vi "WriteFile.vi"(6 "RefreshTime":u32, 7 "Refnum in":T5, 8 "error in (no error)":errorcluster, 9 "BaseMeasurements":T3 {"NHRGridSim Phase" items=["All", "A Phase", "B Phase", "C Phase"]; "NHRDC Measurement Type" items=["Voltage"=1, "Positive Peak Voltage"=2, "Positive Peak Voltage Last Fetch"=4, "Negative Peak Voltage"=8, "Negative Peak Voltage Last Fetch"=16, "Current"=32, "Positive Peak Current"=64, "Positive Peak Current Last Fetch"=128, "Negative Peak Current"=256, "Negative Peak Current Last Fetch"=512, "Power"=1024, "Positive Peak Power"=2048, "Positive Peak Power Last Fetch"=4096, "Negative Peak Power"=8192, "Negative Peak Power Last Fetch"=16384, "Timestamp"=32768, "Charge Time"=65536, "Discharge Time"=131072, "Amp Hour"=262144, "Amp Hour Time"=524288, "Amp Hour Charge"=1048576, "Amp Hour Discharge"=2097152, "Kilo Watt Hour"=4194304, "Kilo Watt Hour Time"=8388608, "Kilo Watt Hour Charge"=16777216, "Kilo Watt Hour Discharge"=33554432, "UUT Temperature"=67108864]; "NHRDC Fetch Method" items=["Aperture", "Immediate"]}, 10 "BaseConfiguration":T1={"Frequency"=0.0, "FrequencyRange"=[], "Phases"=[], "Name"="", "PluginConfigVariant"=variant, "PluginMeasVariant"=variant(cluster{"MeasName":string, "Modules":cluster{"Handle":string, "Connected":bool, "Clear Device (F)":bool, "btnIdQuery":bool, "btnReset":bool, "Program #":cluster{"Phase B (Degrees)":i32, "Waveform A (1: Sine)":i32, "Voltage Level (Va)":dbl, "Program Number (0)":i32, "Voltage Level (Vb) ":dbl, "Form (3: Three)":u16, "Coupling  (0: Direct)":u16, "Frequency (45Hz)":dbl, "Current Limit (40A)":dbl, "Phase C (Degrees)":i32, "Voltage Level (Vc)":dbl, "Waveform B (1: Sine)":i32, "Waveform C (1: Sine)":i32}[], "Impedance Parameters (off, 0.00)":cluster{"State":bool, "Impedance":dbl}, "Transient Execution (F)":bool, "OutputEnabled":bool, "Source Range":cluster{"Frequency Minimum (45 Hz)":dbl, "Frequency Maximum (1200 Hz)":dbl, "Voltage Maximum (V)":dbl, "Voltage Minimum (V)":dbl, "Range Control (0: Auto)":u16, "Initial Voltage (0V)":u16, "Frequency Range (600Hz)":u16}, "Port Type":enum16{"GPIB", "Serial"}}[]} {"MeasName"="", "Modules"=[]})}, 11 "NHRDCModel in":refnum<class "NHRDCModel.lvclass">) -> (0 "error out":errorcluster, 3 "NHRDCModel out":refnum<class "NHRDCModel.lvclass">)   [LabVIEW 2018, in "AcPwrPlugins.lvlib" / "NHRDCModel.lvclass"]
uses:
  NHRDCModel.lvclass
  <vilib>/Utility/config.llb/Config Data RefNum.ctl
  AcPwrBaseClass/TypeDefs/BaseMeasurements.ctl
  ChromaAcLoadClass/TypeDefs/MeasurementType.ctl
  AcPwrBaseClass/TypeDefs/BaseConfig.ctl
  AcPwrBaseClass/TypeDefs/Phase.ctl
  AcPwrBaseClass/AcPwrBase.lvclass
  <vilib>/Utility/config.llb/NI_LVConfig.lvlib
  ChromaAcLoadClass/ChromaAcLoad.lvclass
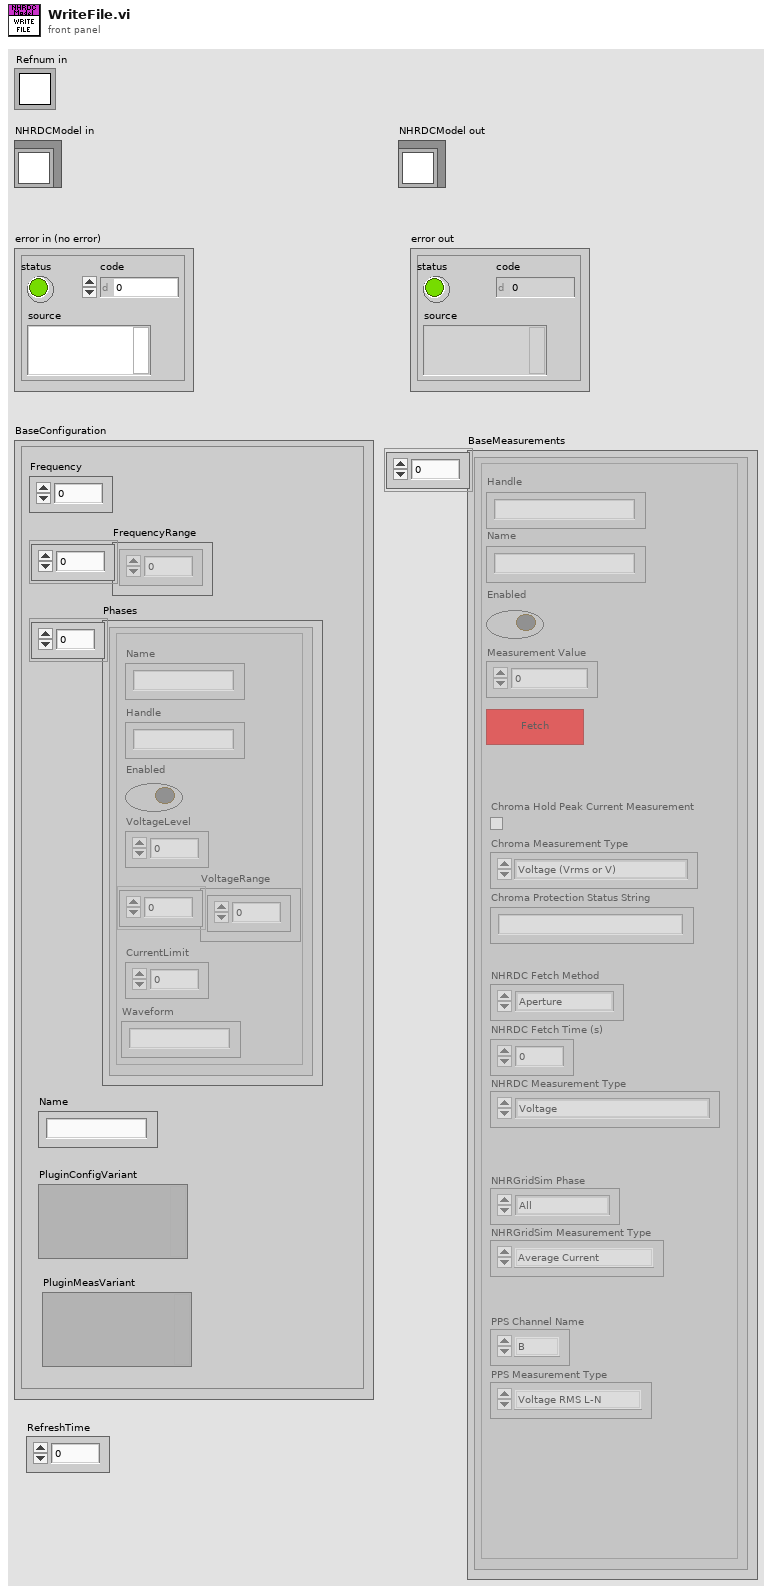
[diagram p1: front panel]
types:
  T1 = typedef "AcPwrPlugins.lvlib/AcPwrBase.lvclass/BaseConfig.ctl" = cluster{"Frequency":dbl, "FrequencyRange":dbl[], "Phases":T2[], "Name":string, "PluginConfigVariant":variant, "PluginMeasVariant":variant}
  T2 = typedef "AcPwrPlugins.lvlib/AcPwrBase.lvclass/Phase.ctl" = cluster{"Name":string, "Enabled":bool, "VoltageLevel":dbl, "Handle":string, "VoltageRange":dbl[], "Connected":bool, "CurrentLimit":dbl, "Waveform":string}
  T3 = typedef "AcPwrPlugins.lvlib/AcPwrBase.lvclass/BaseMeasurements.ctl" = cluster{"Handle":string, "Name":string, "Enabled":bool, "Measurement Value":dbl, "btnMeasFetch":bool, "Chroma Hold Peak Current Measurement":bool, "Chroma Measurement Type":T4, "Chroma Protection Status String":string, "NHRDC Fetch Method":i32, "NHRDC Fetch Time (s)":sgl, "NHRDC Measurement Type":i32, "NHRGridSim Measurement Type ":enum16{"Average Current", "Max Current", "Min Current", "Average Voltage", "Max Voltage", "Min Voltage", "Average True Power", "Max True Power", "Min True Power", "Average Apparent Power", "Max Apparent Power", "Min Apparent Power", "Power Factor", "Crest Factor"}, "NHRGridSim Phase ":i32, "PPS Measurement Type ":enum16{"Voltage RMS L-N", "Voltage RMS L-L", "Frequency", "Current RMS", "Current Peak", "Crest Factor", "Power Factor", "Power VA", "Real Power"}, "PPS Channel Name":enum16{"A", "B", "C"}}[]
  T4 = typedef "AcPwrPlugins.lvlib/ChromaAcLoad.lvclass/MeasurementType.ctl" = enum16{"Voltage (Vrms or V)", "Current (Arms or A)", "Power (W)", "Peak Voltage (V)", "Peak Current (A)", "Peak Power (W)", "Frequency (Hz)", "Resistance (Ohms)", "Voltage Overshoot (V)", "Positive Peak Current (A)", "Voltage Undershoot (V)", "Negative Peak Current (A)", "Apparent Power (VA)", "Reacitive Power (VAR)", "Voltage THD", "Power Factor", "Current's Crest Factor"}
  T5 = typedef "NI_LVConfig.lvlib/Config Data RefNum.ctl" = refnum<k1>
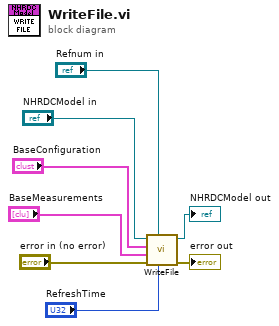
[diagram p0: block diagram]
diagram:
  n1 = call-parent "WriteFile.vi"("RefreshTime"="RefreshTime", "Refnum in"="Refnum in", "error in (no error)"="error in (no error)", "BaseMeasurements"="BaseMeasurements", "BaseConfiguration"="BaseConfiguration", "AcPwrBase in"="NHRDCModel in") -> ("error out"=→"error out":errorcluster, "AcPwrBase out"=→"NHRDCModel out":refnum<class "NHRDCModel.lvclass">)  [unwired: 4 in]
